vi "start_power_measurments.vi"(7 "OphirLMMeasurementLib.ICoLMMeasurement2":refnum<k7>) -> (8 "Power Meter Connection Data Out":T1)   [LabVIEW 2023]
panel:
  out "hDevice":i32
  out "Device S/Ns":string[](array[string])
  out "Selected device S/N":string
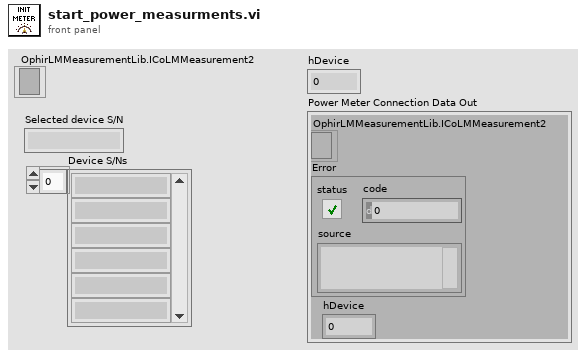
[diagram p1: front panel]
types:
  T1 = cluster{"OphirLMMeasurementLib.ICoLMMeasurement2":refnum<k7>, "Error":errorcluster, "hDevice":i32}
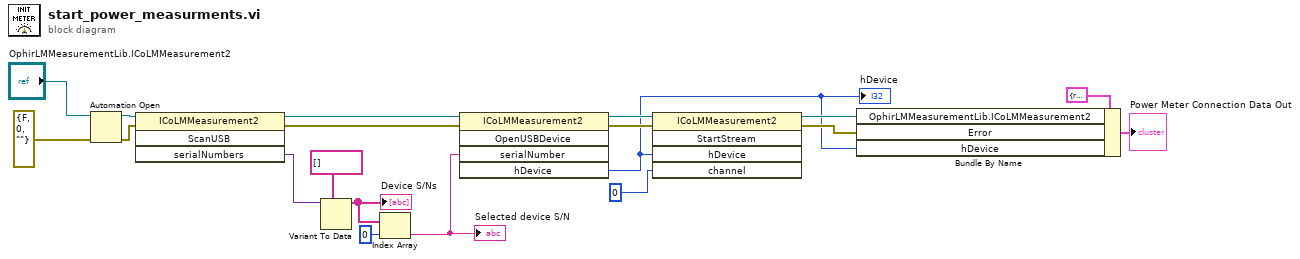
[diagram p0: block diagram]
diagram:
  n1 = Automation Open(error in (no error)=errorcluster {"status"=FALSE, "code"=0, "source"=""}, Automation Refnum="OphirLMMeasurementLib.ICoLMMeasurement2") -> (Automation Refnum=w18:refnum<k7>, error out=w11:errorcluster)  [unwired: 2 in]
  n2 = invoke class="ICoLMMeasurement2" method="ScanUSB"(reference=w18, error in=w11) -> (reference out=w13:refnum<k7>, error out=w12:errorcluster, "serialNumbers"=w17:variant)  [unwired: 2 in, 1 out]
  n3 = Variant To Data(type=string[] [], Variant=w17) -> (data=w16:string[])  [unwired: 1 in, 1 out]
  "Device S/Ns" <- w16
  n4 = Index Array(array=w16, index=0) -> (element=w9:string)
  "Selected device S/N" <- w9
  n5 = invoke class="ICoLMMeasurement2" method="OpenUSBDevice"(reference=w13, error in=w12, "serialNumber"=w9) -> (reference out=w8:refnum<k7>, error out=w7:errorcluster, "hDevice"=w2:i32)  [unwired: 2 in, 2 out]
  "hDevice" <- w2
  n6 = invoke class="ICoLMMeasurement2" method="StartStream"(reference=w8, error in=w7, "hDevice"=w2, "channel"=0) -> (reference out=w4:refnum<k7>, error out=w3:errorcluster)  [unwired: 1 in, 3 out]
  n7 = Bundle By Name(cluster=T1 {"OphirLMMeasurementLib.ICoLMMeasurement2"=refnum, "Error"={"status"=FALSE, "code"=0, "source"=""}, "hDevice"=0}, "OphirLMMeasurementLib.ICoLMMeasurement2"=w4, "Error"=w3, "hDevice"=w2) -> (→"Power Meter Connection Data Out":T1)
